vi "Close.vi"(7 "Abort (F)":bool, 8 "error in (no error)":errorcluster, 11 "Notifier in":refnum<class "Tag.lvclass">) -> (0 "error out":errorcluster)   [LabVIEW 2022 SP3, in "Enclave.lvlib" / "Tag.lvclass"]
uses:
  Tag.lvclass
  Tag.lvclass/Tag.ctl
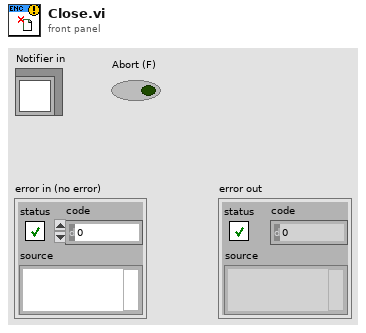
[diagram p1: front panel]
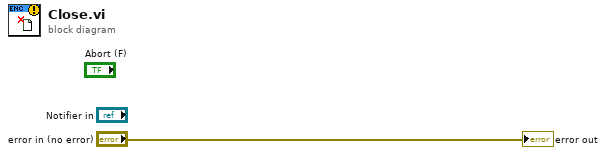
[diagram p0: block diagram]
diagram:
  "error out" <- "error in (no error)"
